vi "Rescue Raw Data.vi"() -> ()   [LabVIEW 2018, in "BinaryTIFF.lvlib" / "TIFF.lvclass"]
uses:
  TIFF.lvclass
panel:
  in  "Duty cycle (fraction)":dbl=1.0 format="%#_13g"
  in  "Camera Model":u16(ring) items=["C11440-22CU", "C13440-20CU", "C14440-20UP", "C15440-20UP", "C15550-20UP"]
  in  "CLOSE":bool
  in  "rescue button":bool
  in  "Horizontal Flip":bool[](array[boolean])=[FALSE, FALSE, FALSE, FALSE]
  in  "Vertical Flip":bool[](array[boolean])=[FALSE, FALSE, FALSE, FALSE]
  in  "Total Frames":u32=101
  in  "Exposure Time (ms)":dbl=100.0
  in  "DCIMG Paths (order: Cy3, Cy5, Cy7, Cy2, unused = blank)":path[](array[path])=[path "", path "", path "", path ""]
  in  "stop":bool=TRUE
  out "Current Frame":i32
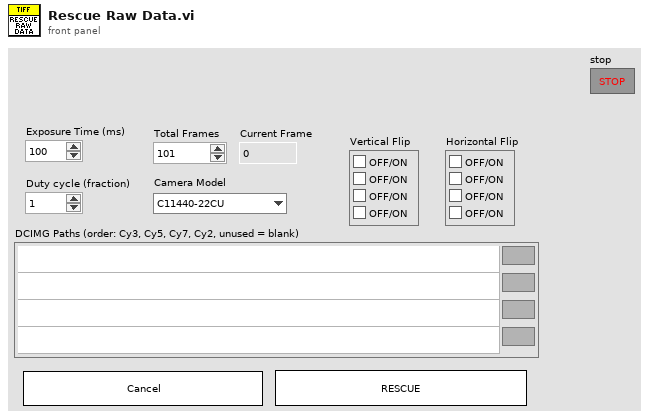
[diagram p1: front panel]
types:
  T1 = enum16{"<unknown>", "Evolve 512", "Orca-Flash 4.0 V2"}
  T2 = enum16{"Open Existing (Read)", "Create or Replace (Write)"}
  T3 = cluster{"Number of Frames":u32, "Image Width (px)":u32, "Image Height (px)":u32, "Pixel Size (nm)":dbl, "Exposure Time (ms)":dbl, "Frame Time (ms)":dbl, "Number of Channels":u32, "Camera Type":enum16{"<unknown>", "Evolve 512", "Orca-Flash 4.0 V2"}, "Bit Depth":u32, "Image Description":string}
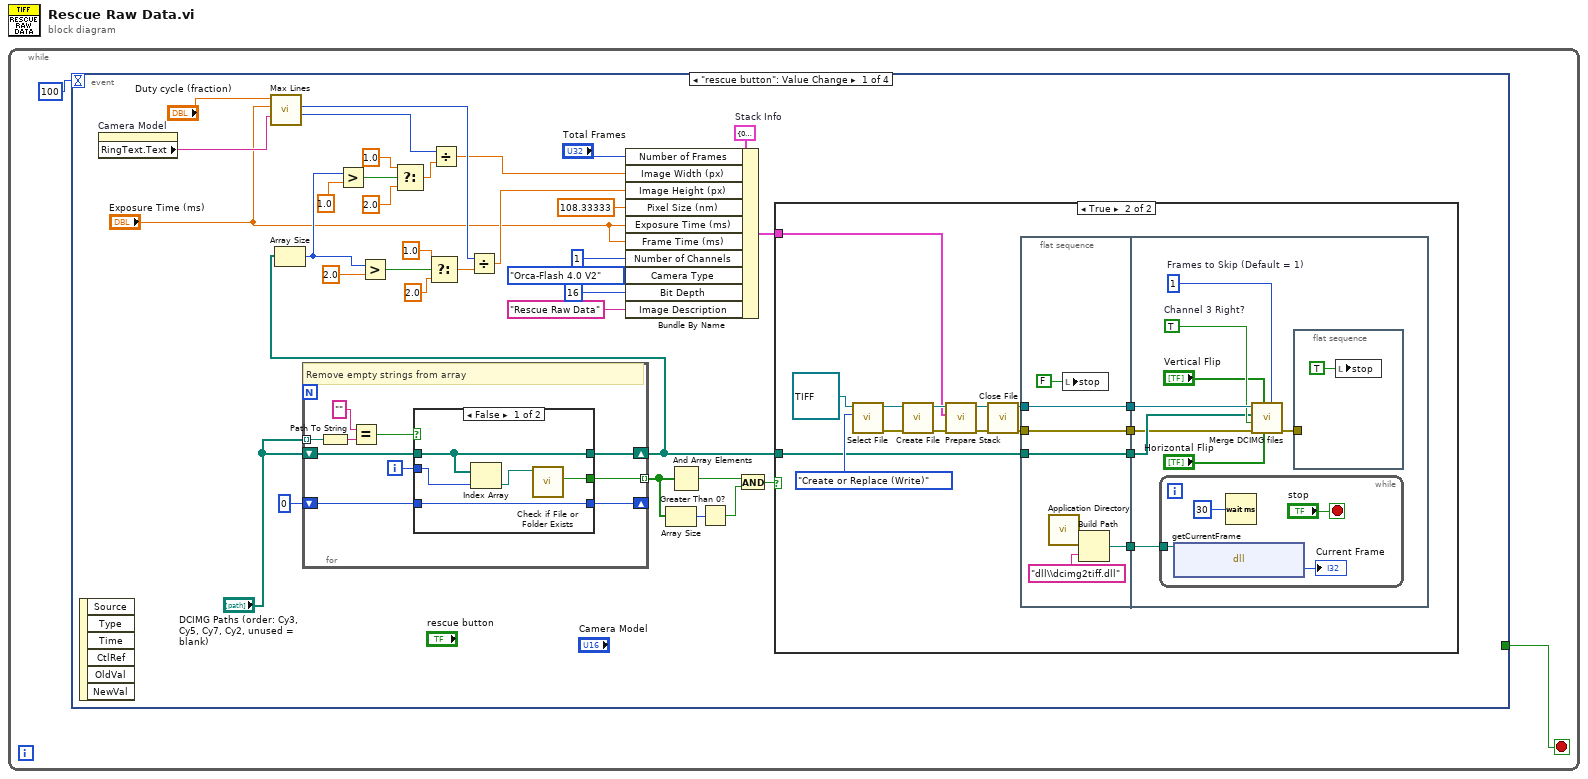
[diagram p0: block diagram]
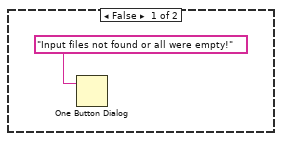
[diagram p2: hidden frame]
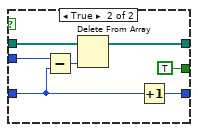
[diagram p3: hidden frame]
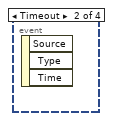
[diagram p4: hidden frame]
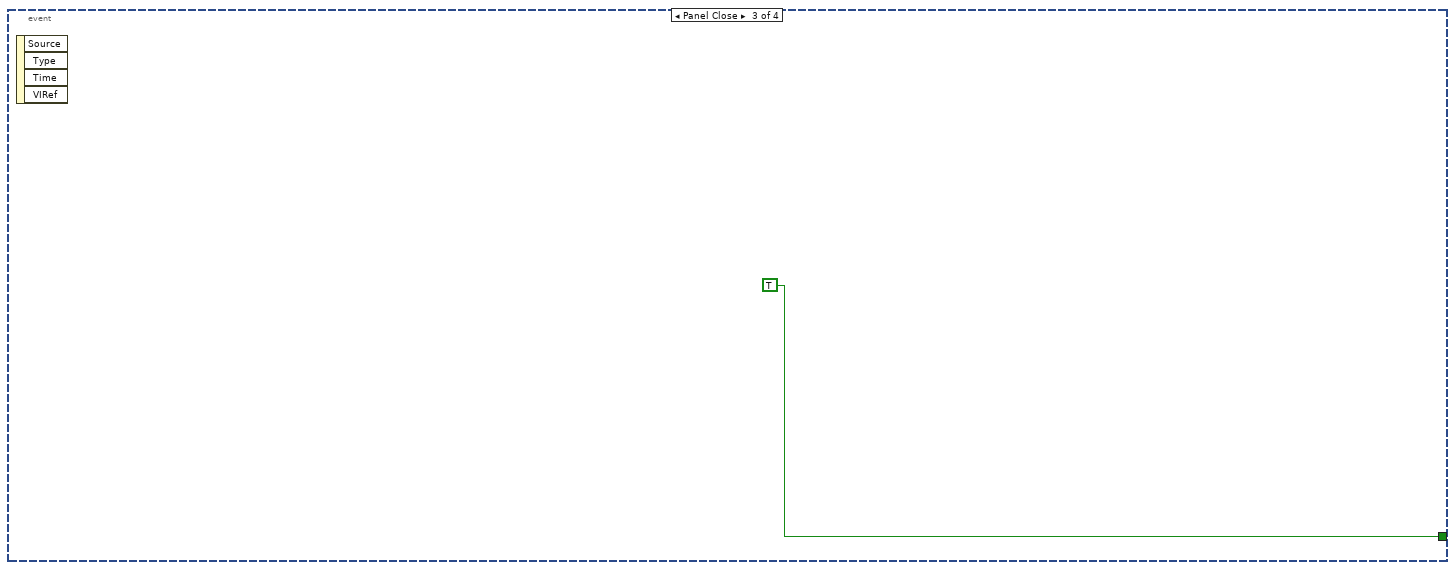
[diagram p5: hidden frame]
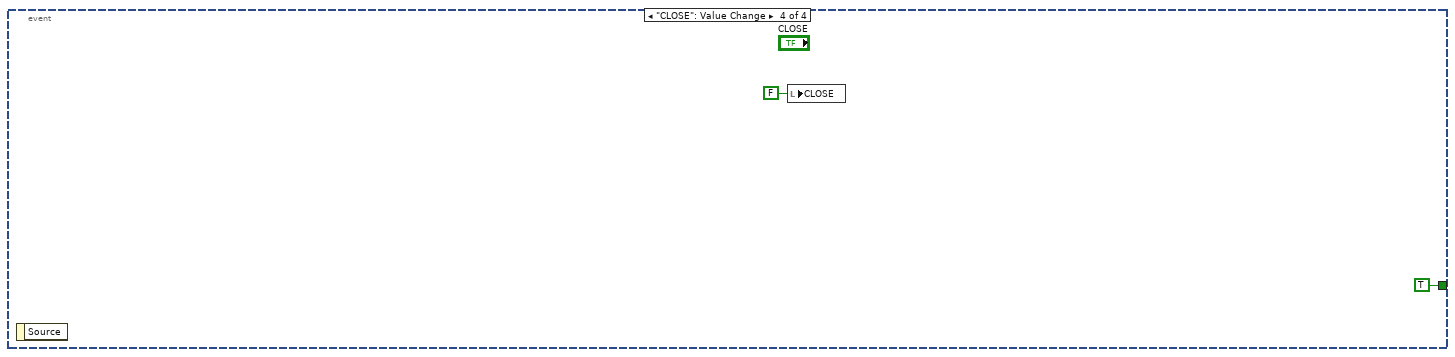
[diagram p6: hidden frame]
diagram:
  n1 = while {
    stop <- w1 stop-if-true
    n2 = event shown="[0] \"rescue button\": Value Change" {
      selector: _ -> [_ _ _ _]
      dyn-events: _ -> [_ _ _ _]
      timeout: 100 -> [_ _ _ _]
      tunnel: [_ _ TRUE ("STOP") TRUE ("STOP")] -> w1
      event "rescue button": Value Change {
        w36 = T3 {"Number of Frames"=0, "Image Width (px)"=0, "Image Height (px)"=0, "Pixel Size (nm)"=0.0, "Exposure Time (ms)"=0.0, "Frame Time (ms)"=0.0, "Number of Channels"=0, "Camera Type"=enum."<unknown>", "Bit Depth"=0, "Image Description"=""}  # Stack Info
        n3 = event-data() -> ()  [unwired: 1 in, 6 out]
        n4 = property on="Camera Model" class="Ring (strict)"() -> ("RingText.Text"=w8:string)  [unwired: 2 in, 2 out]
        n5 = call "Max Lines.vi"("Camera Model"=w8, "Frame Time (ms)"="Exposure Time (ms)", "Duty cycle (fraction)"="Duty cycle (fraction)") -> ("upper limit"=w18:i32, "Max Lines"=w13:i32)  [unwired: 3 in, 4 out]
        n6 = for {
          tunnel: "DCIMG Paths (order: Cy3, Cy5, Cy7, Cy2, unused = blank)" -> [w82] mode=indexing
          shift-right: [w83] -> w4
          shift-left: "DCIMG Paths (order: Cy3, Cy5, Cy7, Cy2, unused = blank)" -> [w84]
          shift-right: [w77] -> _
          shift-left: 0 -> [w76]
          tunnel: [w75] -> w27 mode=indexing
          i -> [w79]
          # "Remove empty strings from array"
          n7 = Path To String(path=w82) -> (string=w81:string)
          n8 = Equal?(x="", y=w81) -> (x = y?=w80:bool)
          n9 = case shown="False" w80 {
            tunnel: w84 -> [w88 w96]
            tunnel: [w88 w95] -> w83
            tunnel: w79 -> [w87 w93]
            tunnel: [w89 w94] -> w77
            tunnel: w76 -> [w89 w92]
            tunnel: [w85 TRUE ("file or folder exists?")] -> w75
            frame False {
              n10 = Index Array(array=w88, index=w87) -> (element=w86:path)
              n11 = call <vilib>:"Check if File or Folder Exists.vi"("path"=w86) -> ("file or folder exists?"=w85:bool)  [unwired: 8 in, 2 out]
            }
            frame True {
              n12 = Subtract(x=w93, y=w92) -> (x-y=w91:i32)
              n13 = Delete From Array(array=w96, index=w91) -> (array with subset deleted=w95:path[])  [unwired: 1 in, 1 out]
              n14 = Increment(x=w92) -> (x+1=w94:i32)
            }
          }
        }
        n15 = Array Size(array=w4) -> (size(s)=w6:i32)
        n16 = Greater?(x=w6, y=1.0) -> (0:w21:bool)
        n17 = Greater?(x=w6, y=2.0) -> (0:w15:bool)
        n18 = Select(t=1.0, s=w21, f=2.0) -> (s? t:f=w17:dbl)
        n19 = Select(t=1.0, s=w15, f=2.0) -> (s? t:f=w14:dbl)
        n20 = Divide(x=w18, y=w17) -> (x/y=w10:dbl)
        n21 = Divide(x=w13, y=w14) -> (x/y=w9:dbl)
        n22 = Bundle By Name(cluster=w36, "Number of Frames"="Total Frames", "Image Width (px)"=w10, "Image Height (px)"=w9, "Pixel Size (nm)"=108.33333, "Exposure Time (ms)"="Exposure Time (ms)", "Frame Time (ms)"="Exposure Time (ms)", "Number of Channels"=u32 1, "Camera Type"=T1."Orca-Flash 4.0 V2", "Bit Depth"=u32 16, "Image Description"="Rescue Raw Data") -> (w32:T3)
        n23 = Array Size(array=w27) -> (size(s)=w26:i32)
        n24 = And Array Elements(Boolean array=w27) -> (logical AND=w24:bool)
        n25 = Greater Than 0?(x=w26) -> (x > 0?=w23:bool)
        n26 = And(x=w24, y=w23) -> (x .and. y?=w25:bool)
        n27 = case shown="True" w25 {
          tunnel: w32 -> [_ w43]
          tunnel: w4 -> [_ w38]
          frame False {
            n28 = One Button Dialog(message="Input files not found or all were empty!") -> ()  [unwired: 1 in, 1 out]
          }
          frame True {
            n29 = call-dynamic "Select File.vi"("Mode"=T2."Create or Replace (Write)", "TIFF in"=refnum<class "TIFF.lvclass"> refnum ("TIFF.lvclass")) -> ("error out"=w46:errorcluster, "TIFF out"=w47:refnum<class "TIFF.lvclass">)  [unwired: 8 in]
            n30 = call-dynamic "Create File.vi"("error in (no error)"=w46, "TIFF in"=w47) -> ("error out"=w44:errorcluster, "TIFF out"=w45:refnum<class "TIFF.lvclass">)  [unwired: 8 in]
            n31 = call-dynamic "Prepare Stack.vi"("error in (no error)"=w44, "Stack Info"=w43, "TIFF in"=w45) -> ("error out"=w41:errorcluster, "TIFF out"=w42:refnum<class "TIFF.lvclass">)  [unwired: 7 in]
            n32 = call-dynamic "Close File.vi"("error in (no error)"=w41, "TIFF in"=w42) -> ("error out"=w39:errorcluster, "TIFF out"=w40:refnum<class "TIFF.lvclass">)  [unwired: 8 in]
            n33 = flat-sequence {
              tunnel: w40 -> [w60]
              tunnel: [w60] -> w53
              tunnel: w38 -> [w58]
              tunnel: [w58] -> w52
              tunnel: [w55] -> w51
              tunnel: [w54] -> w50
              tunnel: w39 -> [w54]
              tunnel: w53 -> [w69]
              tunnel: w52 -> [w65]
              tunnel: w51 -> [w64]
              tunnel: w50 -> [w62]
              frame #0 {
                n34 = call <vilib>:"Application Directory.vi"() -> ("Application Directory"=w56:path)
                n35 = local write "stop"(FALSE ("stop")) -> ()
                n36 = Build Path(base path=w56, name or relative path="dll\\dcimg2tiff.dll") -> (appended path=w55:path)
              }
              frame #1 {
                w61 = u32 1  # Frames to Skip (Default = 1)
                w66 = TRUE  # Channel 3 Right?
                n37 = while {
                  tunnel: w64 -> [w71]
                  stop <- "stop" stop-if-true
                  n38 = dll-call lib="?" fn="getCurrentFrame"(path in=w71) -> ("Current Frame"=→"Current Frame":u64)  [unwired: 2 in, 2 out]
                  n39 = Wait (ms)(milliseconds to wait=u32 30) -> ()  [unwired: 1 out]
                }
                n40 = call-dynamic "Merge DCIMG files.vi"("Frames to Skip"=w61, "Horizontal Flip"="Horizontal Flip", "Vertical Flip"="Vertical Flip", "error in (no error)"=w62, "Channel 3 Right?"=w66, "DCIMG Paths (2 to 4)"=w65, "TIFF in"=w69) -> ("error out"=w68:errorcluster)  [unwired: 3 in, 1 out]
                n41 = flat-sequence {
                  tunnel: w68 -> [_]
                  frame #0 {
                    n42 = local write "stop"(TRUE ("stop")) -> ()
                  }
                }
              }
            }
          }
        }
      }
      event Timeout {
        n43 = event-data() -> ()  [unwired: 1 in, 3 out]
      }
      event Panel Close {
        n44 = event-data() -> ()  [unwired: 1 in, 4 out]
      }
      event "CLOSE": Value Change {
        n45 = event-data() -> ()  [unwired: 1 in, 1 out]
        n46 = local write "CLOSE"(FALSE ("CLOSE")) -> ()
      }
    }
  }
